vi "Coherent Output Power.vi"(0 "scaled signal X [EUx]":dbl[](array[numeric]) format="%.2f", 1 "scaled signal Y [EUy]":dbl[](array[numeric]) format="%.2f", 2 "sampling frequency [Hz]":dbl=10000.0 format="%.2f", 3 "dB On (F)":bool, 5 "channel Y info":T2={"sensor sensitivity [mV/EU]"=1000.0, "engineering units"=1, "dB reference [EU]"=1.0, "custom label"="EU", "weighting filter"=0, "pregain [dB]"=0.0} {"pregain [dB]" format="%.2f"; "weighting filter" items=["Linear", "A-weighting", "B-weighting", "C-weighting", "ITU-R 468-4", "Dolby", "CCITT", "C-message"]; "dB reference [EU]" format="%^.1e"; "engineering units" items=["custom..."=0, "V"=1, "A"=21, "Pa"=2, "N"=20, "g"=3, "m/s^2"=4, "m/s"=5, "m"=6, "mm/s"=12, "mm"=13, "microns/s"=14, "microns"=15, "in/s^2"=7, "in/s"=8, "in"=9, "mils/s"=10, "mils"=11, "rad/s^2"=16, "rad/s"=17, "rad"=18, "strain"=19]; "sensor sensitivity [mV/EU]" format="%.2f"}, 6 "window":T6=1 items=["None"=0, "Hanning"=1, "Hamming"=2, "Blackman-Harris"=3, "Exact Blackman"=4, "Blackman"=5, "Flat Top"=6, "4 Term B-Harris "=7, "7 Term B-Harris"=8, "Low Sidelobe"=9, "Force - Exponential"=10, "Blackman Nuttall"=11, "Triangle"=30, "Bartlett-Hanning"=31, "Bohman"=32, "Parzen"=33, "Welch"=34, "Kaiser"=60, "Dolph-Chebyshev"=61, "Gaussian"=62], 7 "reset averaging (T)":bool=TRUE, 8 "force/exp settings":T5={"force window [%]"=50.0, "exponential window [%]"=10.0} {"exponential window [%]" min=0.0 max=100.0 format="%.2f"; "force window [%]" min=0.0 max=100.0 format="%.2f"}, 9 "averaging parameters":T1={"averaging mode"=enum."RMS averaging", "weighting mode"=enum."Linear", "number of averages"=10} {"number of averages" min=1}) -> (13 "window constants":cluster{"eq noise BW":dbl, "coherent gain":dbl} {"coherent gain" format="%.2f"; "eq noise BW" format="%.2f"}, 14 "coherent output power [EUy^2 rms]":dbl[](array[numeric]) format="%.2f", 15 "unit label":string, 16 "coherence":dbl[](array[numeric]) format="%.2f", 17 "df [Hz]":dbl format="%.2f", 18 "averages completed":dbl format="%.2f", 19 "error out":errorcluster)   [LabVIEW 2017]
doc: "Computes the coherent output power and the coherence based on the input signals. \nTypically, X signal is the stimulus and Y signal is the response of the system.\nCoherent output power is typically an averaged measurement. Each block of data corresponds to a single FFT block and must be passed individually to this VI. The first time this VI is called, reset averaging must be TRUE (default value), to start a new averaging process. For subsequent calls, reset averaging must be FALSE to continue the averaging process. Averages completed returns the number of averages completed so far.\nAveraging parameters specifies how the averaging is performed. The only available averaging mode is RMS averaging. Other parameters include the weighting mode (linear or exponential) and the number of averages (used only if the weighting mode is exponential)."
uses:
  <vilib>/addons/_NISVFA/_Shared subVIs/Controls/svc_Window [Dual FFT].ctl
  <vilib>/addons/Sound and Vibration/compatibility/Controls/svl_Channel Info.ctl
  <vilib>/addons/Sound and Vibration/compatibility/Controls/svl_Engineering Units Text Ring.ctl
  <vilib>/addons/Sound and Vibration/compatibility/Controls/svl_Weighting Filter Text Ring.ctl
  <vilib>/Analysis/4window.llb/Force Window (DBL).vi
  <vilib>/Analysis/4window.llb/Exponential Window (DBL).vi
  <vilib>/Analysis/2dsp.llb/Power Spectrum (DBL).vi
  <vilib>/Analysis/2dsp.llb/Cross Power (DBL).vi
  <vilib>/Analysis/0measdsp.llb/Scaled Time Domain Window (DBL).vi
  <vilib>/Analysis/NI_AALPro.lvlib
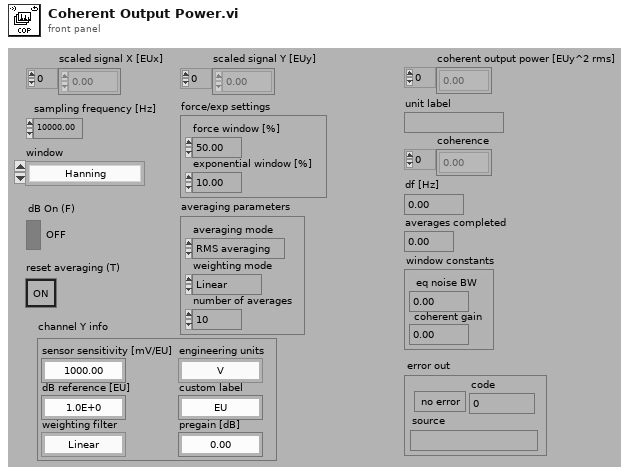
[diagram p1: front panel]
types:
  T1 = cluster{"averaging mode":enum16{"RMS averaging"}, "weighting mode":enum16{"Linear", "Exponential"}, "number of averages":u32}
  T2 = typedef "svl_Channel Info.ctl" = cluster{"sensor sensitivity [mV/EU]":dbl, "engineering units":T3, "dB reference [EU]":dbl, "custom label":string, "weighting filter":T4, "pregain [dB]":dbl}
  T3 = typedef "svl_Engineering Units Text Ring.ctl" = u16
  T4 = typedef "svl_Weighting Filter Text Ring.ctl" = u16
  T5 = cluster{"force window [%]":dbl, "exponential window [%]":dbl}
  T6 = typedef "svc_Window [Dual FFT].ctl" = u32
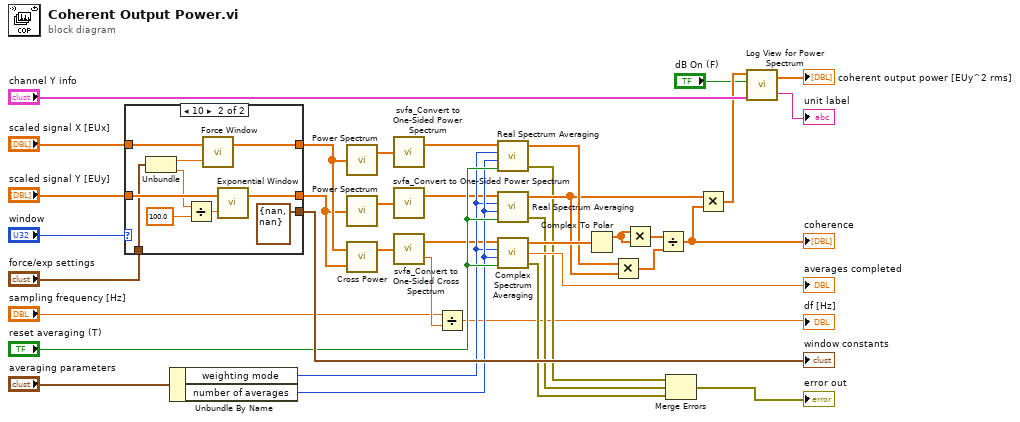
[diagram p0: block diagram]
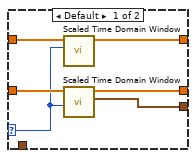
[diagram p2: hidden frame]
diagram:
  n1 = case shown="10" "window" {
    selector: "window" -> [w38 _]
    tunnel: "scaled signal X [EUx]" -> [w43 w53]
    tunnel: "scaled signal Y [EUy]" -> [w42 w52]
    tunnel: "force/exp settings" -> [_ w48]
    tunnel: [w41 w50] -> w4
    tunnel: [w40 w49] -> w2
    tunnel: [w39 cluster{"eq noise BW":dbl, "coherent gain":dbl} {"eq noise BW"=nan, "coherent gain"=nan} ("window constants")] -> w35
    frame Default {
      n2 = call-poly <vilib>:"Scaled Time Domain Window.vi"("window"=w38, "X"=w43) -> ("Windowed X"=w41:dbl[])  [unwired: 7 in, 2 out]
      n3 = call-poly <vilib>:"Scaled Time Domain Window.vi"("window"=w38, "X"=w42) -> ("window properties"=w39:cluster{"eq noise BW":dbl, "coherent gain":dbl}, "Windowed X"=w40:dbl[])  [unwired: 7 in, 1 out]
    }
    frame 10 {
      n4 = Unbundle(w48) -> ("force window [%]"=w47:dbl, "exponential window [%]"=w46:dbl)
      n5 = Divide(x=w46, y=100.0 ("x")) -> (x/y=w51:dbl)
      n6 = call-poly <vilib>:"Force Window.vi"("duty cycle(%)"=w47, "X"=w53) -> ("Windowed X"=w50:dbl[])  [unwired: 1 out]
      n7 = call-poly <vilib>:"Exponential Window.vi"("final value"=w51, "X"=w52) -> ("Windowed X"=w49:dbl[])  [unwired: 1 out]
    }
  }
  "window constants" <- w35
  n8 = Unbundle By Name("averaging parameters") -> ("weighting mode"=w16:enum16{"Linear", "Exponential"}, "number of averages"=w17:u32)
  n9 = call-poly <vilib>:"Power Spectrum.vi"("X"=w4) -> ("Power Spectrum"=w6:dbl[])  [unwired: 1 out]
  n10 = call-poly <vilib>:"Power Spectrum.vi"("X"=w2) -> ("Power Spectrum"=w5:dbl[])  [unwired: 1 out]
  n11 = call-poly <vilib>:"Cross Power.vi"("Y"=w2, "X"=w4) -> ("Sxy"=w11:cdb[])  [unwired: 1 out]
  n12 = call <vilib>:"svfa_Convert to One-Sided Power Spectrum.vi"("two-sided power spectrum"=w6) -> ("one-sided power spectrum"=w3:dbl[])  [unwired: 1 out]
  n13 = call <vilib>:"svfa_Convert to One-Sided Power Spectrum.vi"("two-sided power spectrum"=w5) -> ("one-sided power spectrum"=w1:dbl[])  [unwired: 1 out]
  n14 = call <vilib>:"svfa_Convert to One-Sided Cross Spectrum.vi"("two-sided cross spectrum"=w11) -> ("one-sided cross spectrum"=w9:cdb[], "block size"=w10:dbl)
  n15 = Divide(x="sampling frequency [Hz]", y=w10) -> (x/y=→"df [Hz]":dbl)
  n16 = call <vilib>:"Real Spectrum Averaging.vi"("reset averaging (T)"="reset averaging (T)", "number of averages"=w17, "weighting mode"=w16, "real spectrum"=w3) -> ("error out"=w15:errorcluster, "averaged real spectrum"=w27:dbl[])  [unwired: 1 out]
  n17 = call <vilib>:"Real Spectrum Averaging.vi"("reset averaging (T)"="reset averaging (T)", "number of averages"=w17, "weighting mode"=w16, "real spectrum"=w1) -> ("error out"=w14:errorcluster, "averaged real spectrum"=w26:dbl[])  [unwired: 1 out]
  n18 = call <vilib>:"Complex Spectrum Averaging.vi"("reset averaging (T)"="reset averaging (T)", "number of averages"=w17, "weighting mode"=w16, "complex spectrum"=w9) -> ("error out"=w13:errorcluster, "averages completed"=→"averages completed":dbl, "averaged complex spectrum"=w31:cdb[])
  n19 = Complex To Polar(r * e^(i*theta)=w31) -> (r=w28:dbl[])  [unwired: 1 out]
  n20 = Multiply(x=w27, y=w26) -> (x*y=w29:dbl[])
  n21 = Multiply(x=w28, y=w28) -> (x*y=w30:dbl[])
  n22 = Divide(x=w30, y=w29) -> (x/y=w25:dbl[])
  "coherence" <- w25
  n23 = Merge Errors(w15, w14, w13) -> (→"error out":errorcluster)
  n24 = Multiply(x=w26, y=w25) -> (x*y=w23:dbl[])
  n25 = call <vilib>:"Log View for Power Spectrum.vi"("channel info"="channel Y info", "dB On (T)"="dB On (F)", "power spectrum [EU^2 rms]"=w23) -> ("unit label"=→"unit label":string, "log view power spectrum [dB EU]"=→"coherent output power [EUy^2 rms]":dbl[])  [unwired: 1 in]
